vi "Send 2_Subscribe.vi"(7 "Priority":T3=enum."Normal" caption="Message Priority (Normal)", 8 "error in (no error)":errorcluster, 10 "Subscribe":T1, 11 "Message Enqueuer in":refnum<class "Message Enqueuer.lvclass">) -> (0 "error out":errorcluster, 3 "Message Enqueuer out":refnum<class "Message Enqueuer.lvclass">)   [LabVIEW 2018, in "MQTT_Client_Actor.lvlib" / "2_Subscribe Msg.lvclass"]
doc: "Sends the <b>MQTT_Client_Actor.lvlib:2_Subscribe Msg.lvclass</b> message.\n\nThis message will call <b>2_Subscribe.vi</b> on the <b>MQTT_Client_Actor.lvlib:MQTT_Client_Actor.lvclass</b> actor.\n\n<b>2_Subscribe.vi Description</b>"
uses:
  2_Subscribe Msg.lvclass
  <vilib>/ActorFramework/Message Enqueuer/Message Enqueuer.lvclass
  <vilib>/ActorFramework/Message Enqueuer/Message Priority.ctl
  MQTT_Client_Actor/SubscribeClient.ctl
  <vilib>/LabVIEW Open Source Project/MQTT Control Packets/Control Packets/ControlPacket/QualityOfService -- enum.ctl
  D:/Program Files (x86)/National Instruments/LabVIEW 2018/vi.lib/ActorFramework/Message/Message.lvclass
  2_Subscribe Msg.lvclass/2_Subscribe Msg.ctl
  <vilib>/ActorFramework/Message Enqueuer/Message Enqueuer.lvclass/Message Enqueuer.ctl
  <vilib>/ActorFramework/Message Priority Queue/Priority Enqueue.vi
  <vilib>/LabVIEW Open Source Project/MQTT Control Packets/Control Packets/ControlPacket/ControlPacket.lvclass
  MQTT_Client_Actor/MQTT_Client_Actor.lvclass
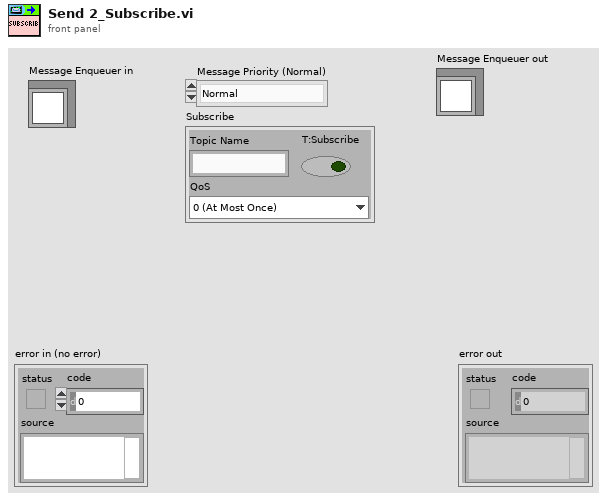
[diagram p1: front panel]
types:
  T1 = typedef "MQTT_Client_Actor.lvlib/MQTT_Client_Actor.lvclass/SubscribeClient.ctl" = cluster{"Topic Name":string, "QoS":T2, "T:Subscribe":bool}
  T2 = typedef "MQTT_Control_Packets.lvlib/ControlPacket.lvclass/QualityOfService -- enum.ctl" = enum16{"0 (At Most Once)", "1 (At Least Once)", "2 (Exactly Once)"}
  T3 = typedef "Actor Framework.lvlib/Message Enqueuer.lvclass/Message Priority.ctl" = enum16{"Low", "Normal", "High"}
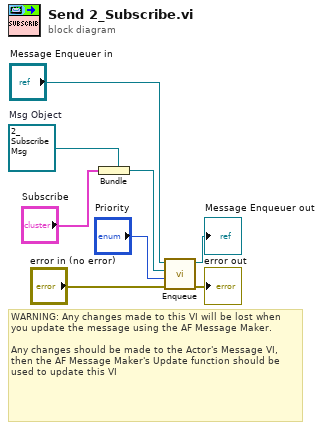
[diagram p0: block diagram]
diagram:
  w7 = refnum<class "2_Subscribe Msg.lvclass"> refnum  # Msg Object
  # "WARNING: Any changes made to this VI will be lost when you update the message using the AF Message Maker.\n\nAny changes should be made to the Actor's Message VI, then the AF Message Maker's Update function should be used to update this VI"
  n1 = Bundle(cluster=w7, "Subscribe") -> (w2:refnum<class "2_Subscribe Msg.lvclass">)
  n2 = call <vilib>:"Enqueue.vi"("error in (no error)"="error in (no error)", "Message Priority (Normal)"="Priority", "Message"=w2, "Message Enqueuer in"="Message Enqueuer in") -> ("error out"=→"error out":errorcluster, "Message Enqueuer out"=→"Message Enqueuer out":refnum<class "Message Enqueuer.lvclass">)  [unwired: 6 in]
